vi "Tree Structures.vi"() -> ()   [LabVIEW 2022 SP3]
panel:
  out "Map":T1(c390)
  out "Array":T2(array[cluster])
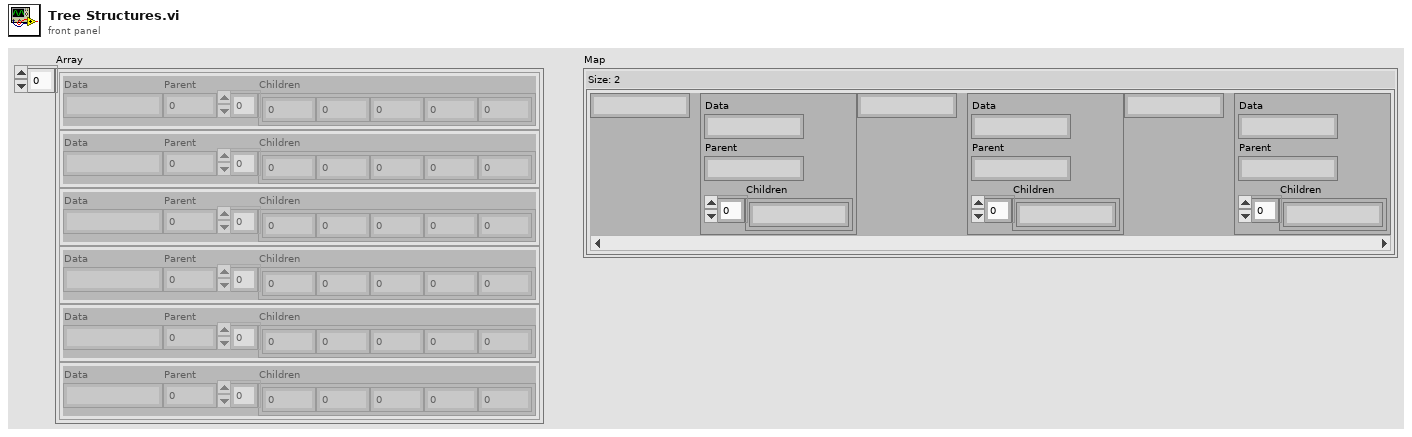
[diagram p1: front panel]
types:
  T1 = map{string, cluster{"Data":string, "Parent":string, "Children":string[]}}
  T2 = cluster{"Data":string, "Parent":i32, "Children":i32[]}[]
  T3 = cluster{"Data":string, "Parent":string, "Children":string[]}
  T4 = cluster{"Data":string, "Parent":i32, "Children":i32[]}
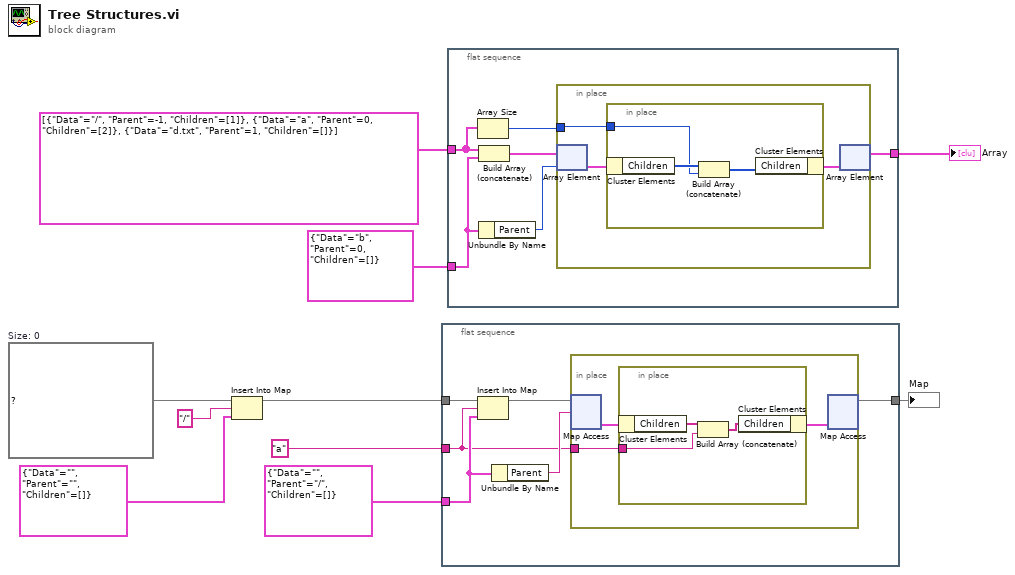
[diagram p0: block diagram]
diagram:
  w7 = T1 {}  # Size: 0
  n1 = Insert Into Map(map in=w7, key="/", value=T3 {"Data"="", "Parent"="", "Children"=[]}) -> (map out=w4:T1)  [unwired: 2 out]
  n2 = flat-sequence {
    tunnel: w4 -> [w16]
    tunnel: "a" -> [w12]
    tunnel: T3 {"Data"="", "Parent"="/", "Children"=[]} -> [w14]
    tunnel: [w11] -> w1
    frame #0 {
      n3 = Insert Into Map(map in=w16, key=w12, value=w14) -> (map out=w15:T1)  [unwired: 2 out]
      n4 = Unbundle By Name(w14) -> ("Parent"=w13:string)
      n5 = in-place {
        in-place-border: w12 -> [w18]
        n6 = in-place-map #1(w15, w13) -> (w19:T3)  [unwired: 1 in, 1 out]
        n7 = in-place {
          in-place-border: w18 -> [w21]
          n8 = in-place-cluster #2(w19) -> ("Children"=w22:string[])
          n9 = Build Array (concatenate)(w22, w21) -> (w20:string[])
          n10 = in-place-cluster #2("Children"=w20) -> (w17:T3)
        }
        n11 = in-place-map #1(w17) -> (w11:T1)  [unwired: 1 in, 2 out]
      }
    }
  }
  n12 = flat-sequence {
    tunnel: T4 {"Data"="b", "Parent"=0, "Children"=[]} -> [w28]
    tunnel: T2 [{"Data"="/", "Parent"=-1, "Children"=[1]}, {"Data"="a", "Parent"=0, "Children"=[2]}, {"Data"="d.txt", "Parent"=1, "Children"=[]}] -> [w27]
    tunnel: [w23] -> w8
    frame #0 {
      n13 = Array Size(array=w27) -> (size(s)=w26:i32)
      n14 = Build Array (concatenate)(w27, w28) -> (w25:T2)
      n15 = Unbundle By Name(w28) -> ("Parent"=w24:i32)
      n16 = in-place {
        in-place-border: w26 -> [w30]
        n17 = in-place-array #3(w25, w24) -> (w31:T4)
        n18 = in-place {
          in-place-border: w30 -> [w33]
          n19 = in-place-cluster #4(w31) -> ("Children"=w34:i32[])
          n20 = Build Array (concatenate)(w34, w33) -> (w32:i32[])
          n21 = in-place-cluster #4("Children"=w32) -> (w29:T4)
        }
        n22 = in-place-array #3(w29) -> (w23:T2)  [unwired: 1 out]
      }
    }
  }
  "Array" <- w8
  "Map" <- w1
